vi "Cube Drop.vi"   [LabVIEW 2020, in "VolatusSeqGUI.lvlib"]
uses:
  VolatusSeqGUI.lvlib
  Sequencing Control/Sequencing Control.lvclass
  VolatusSeqConfig/VolatusSeqConfig.lvlib
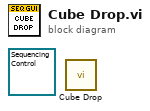
[diagram p0: block diagram]
diagram:
  (unwired) refnum<class "Sequencing Control.lvclass"> refnum ("VolatusSeqGUI.lvlib:Sequencing Control.lvclass")
  n1 = call "Cube Drop.vi"() -> ()  [unwired: 12 in]
